vi "calc_curve averaging.vi"(8 "error in (no error)":errorcluster, 10 "DAQ Read Array":dbl[][](array[numeric])) -> (0 "error out":errorcluster, 1 "Consumed Time(ms)":u32, 2 "Curve (Averaged)":dbl[](array[numeric]))   [LabVIEW 2016]
uses:
  <vilib>/gmath/NI_Gmath.lvlib
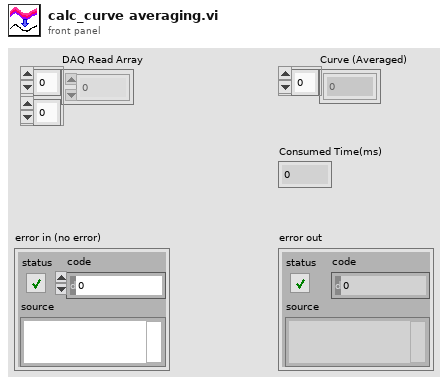
[diagram p1: front panel]
types:
  T1 = enum16{"arithmetic", "geometric", "harmonic", "trimmed", "median"}
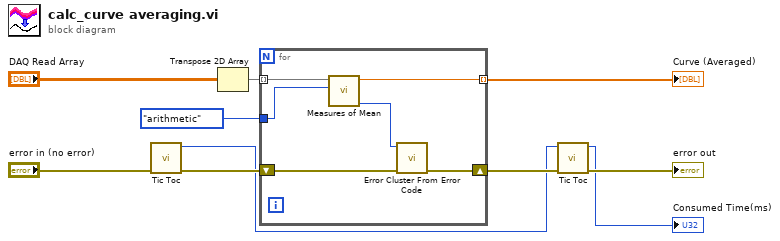
[diagram p0: block diagram]
diagram:
  n1 = call "Tic Toc.vi"("error in (no error)"="error in (no error)") -> ("error out"=w3:errorcluster, "New Toc"=w1:u32)  [unwired: 8 in, 1 out]
  n2 = Transpose 2D Array(2D array="DAQ Read Array") -> (transposed array=w10:dbl[][])
  n3 = for {
    tunnel: w10 -> [w16] mode=indexing
    tunnel: [w15] -> w7 mode=indexing
    tunnel: T1."arithmetic" ("type") -> [w14]
    shift-right: [w13] -> w6
    shift-left: w3 -> [w12]
    n4 = call <vilib>:"Measures of Mean.vi"("type"=w14, "x array"=w16) -> ("error"=w11:i32, "mean value"=w15:dbl)  [unwired: 8 in]
    n5 = call <vilib>:"Error Cluster From Error Code.vi"("error in (no error)"=w12, "error code (0)"=w11) -> ("error out"=w13:errorcluster)  [unwired: 7 in]
  }
  "Curve (Averaged)" <- w7
  n6 = call "Tic Toc.vi"("error in (no error)"=w6, "Last Tic"=w1) -> ("error out"=→"error out":errorcluster, "New Toc"=→"Consumed Time(ms)":u32)  [unwired: 7 in, 1 out]
